vi "Pointer producer consumer autobalance.vi"(9 "Real-time Values":dbl[](array[numeric]), 11 "Auto Balance":bool=TRUE) -> (1 "New ADC Values":dbl[](array[numeric]), 3 "AB Active":bool=TRUE)   [LabVIEW 2014]
panel:
  out "New ADC2":dbl
  out "New ADC3":dbl
  out "ADC2":dbl
  out "ADC3":dbl
  out "ADC0-ADC2":dbl
  out "ADC1-ADC3":dbl
  out "ADC3":dbl
  out "ADC2":dbl
  out "ADC1":dbl
  out "ADC0":dbl
  # "Real Time Values"
  # "Difference of Frozen Values"
  # "New Values"
  # "Frozen Values"
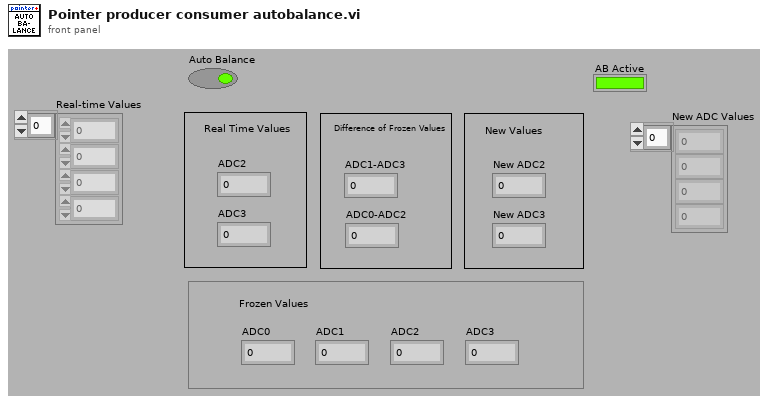
[diagram p1: front panel]
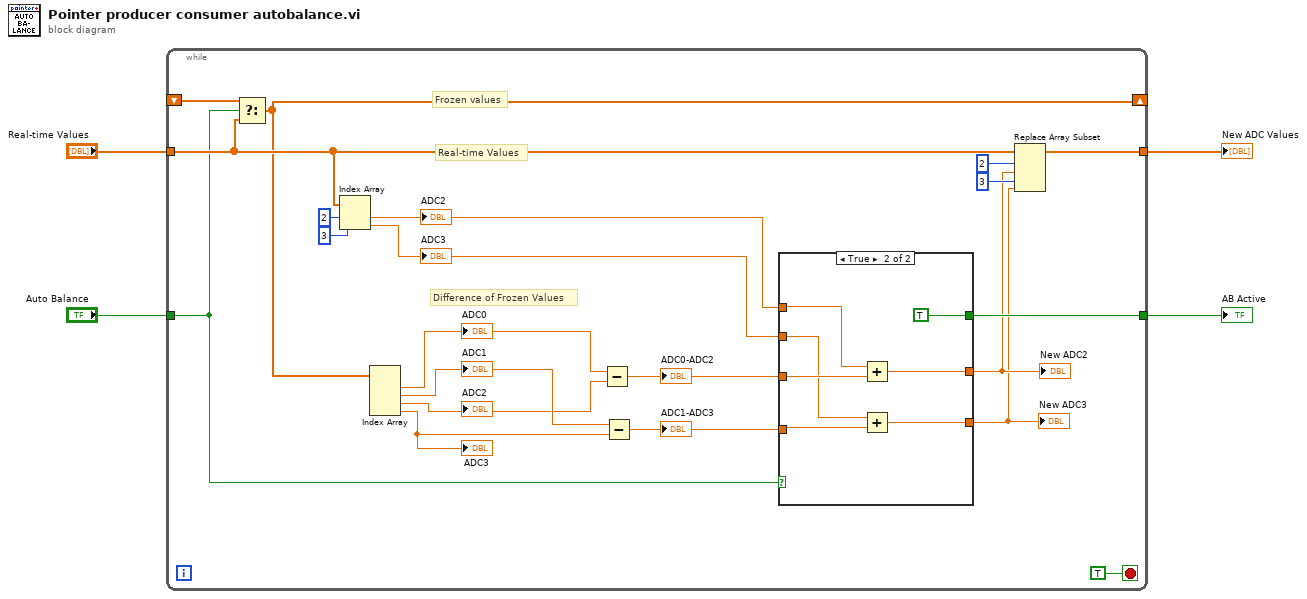
[diagram p0: block diagram]
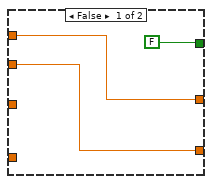
[diagram p2: hidden frame]
diagram:
  n1 = while {
    tunnel: "Real-time Values" -> [w8]
    tunnel: [w17] -> w1
    tunnel: "Auto Balance" -> [w6]
    tunnel: [w22] -> w4
    shift-right: [w7] -> _
    shift-left: _ -> [w9]
    stop <- TRUE stop-if-true
    # "Real-time Values"
    # "Frozen values"
    # "Difference of Frozen Values"
    n2 = Select(t=w9, s=w6, f=w8) -> (s? t:f=w7:dbl[])
    n3 = Index Array(array=w8, index #1=2 ("index"), index #2=3 ("index")) -> (element #1=w19:dbl, element #2=w18:dbl)
    "ADC3" <- w18
    "ADC2" <- w19
    n4 = Index Array(array=w7) -> (element #1=w25:dbl, element #2=w12:dbl, element #3=w11:dbl, element #4=w10:dbl)  [unwired: 4 in]
    "ADC0" <- w25
    "ADC1" <- w12
    "ADC2" <- w11
    "ADC3" <- w10
    n5 = Subtract(x=w25, y=w11) -> (x-y=w24:dbl)
    "ADC0-ADC2" <- w24
    n6 = Subtract(x=w12, y=w10) -> (x-y=w23:dbl)
    "ADC1-ADC3" <- w23
    n7 = case shown="True" w6 {
      tunnel: w24 -> [_ w34]
      tunnel: w23 -> [_ w32]
      tunnel: w19 -> [w28 w35]
      tunnel: w18 -> [w27 w33]
      tunnel: [w28 w31] -> w14
      tunnel: [w27 w30] -> w13
      tunnel: [FALSE TRUE] -> w22
      frame False {
      }
      frame True {
        n8 = Add(x=w35, y=w34) -> (x+y=w31:dbl)
        n9 = Add(x=w33, y=w32) -> (x+y=w30:dbl)
      }
    }
    "New ADC2" <- w14
    "New ADC3" <- w13
    n10 = Replace Array Subset(array=w8, new element #1=w14, index #1=2 ("index"), new element #2=w13, index #2=3 ("index")) -> (w17:dbl[])
  }
  "AB Active" <- w4
  "New ADC Values" <- w1
